vi "PolynomialSegmentScalar.vi"(5 "msg in":string) -> (2 "msg out":string)   [LabVIEW 2018]
doc: "Flattens an float64 scaler into a message"
uses:
  <userlib>/ROS for LabVIEW Software/ROS/MessageBuilding/std_msgs/subs/i32Scalar.vi
  <userlib>/ROS for LabVIEW Software/ROS/MessageBuilding/std_msgs/subs/durationScalar.vi
  <userlib>/ROS for LabVIEW Software/ROS/MessageBuilding/std_msgs/subs/float64Array.vi
panel:
  in  "degree":i32
  in  "Duration":cluster{"secs":i32, "nsecs":i32}
  in  "coefs":dbl[](array[numeric])
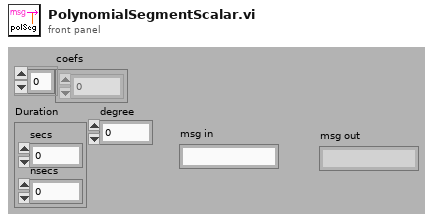
[diagram p1: front panel]
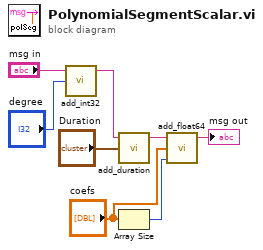
[diagram p0: block diagram]
diagram:
  n1 = call-poly <userlib>:"add_int32.vi"("Numeric"="degree", "msg in"="msg in") -> ("msg out"=w3:string)  [unwired: 3 in]
  n2 = call-poly <userlib>:"add_duration.vi"("Duration"="Duration", "msg in"=w3) -> ("msg out"=w2:string)  [unwired: 3 in]
  n3 = Array Size(array="coefs") -> (size(s)=w7:i32)
  n4 = call-poly <userlib>:"add_float64.vi"("Array Length"=w7, "Array"="coefs", "msg in"=w2) -> ("msg out"=→"msg out":string)  [unwired: 2 in]
